vi "Steps Handler.vi"(7 "Operation":enum16{"Setup", "Next State"}(ring), 9 "Zone Setup Array":cluster{"Zone Selector":string, "Timing":dbl}[](array[cluster]), 10 "Run Selector":bool) -> (2 "Next State":cluster{"Value":T1, "Timing":dbl})   [LabVIEW 2025]
uses:
  Controls/States.ctl
panel:
  out "Array 2":cluster{"Value":T1, "Timing":dbl}[](array[cluster])
  out "Array":cluster{"Value":T1, "Timing":dbl}[](array[cluster])
  in  "State":T1
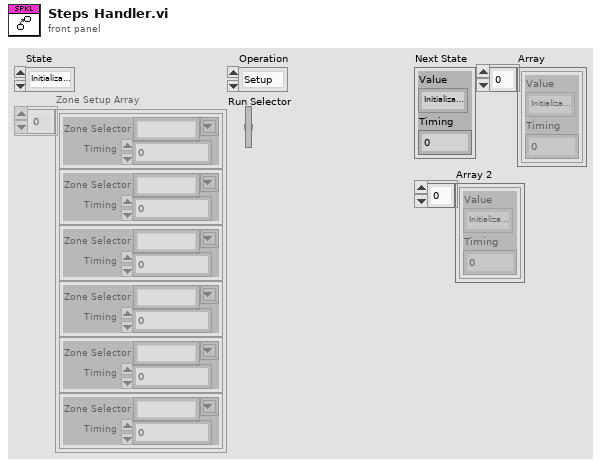
[diagram p1: front panel]
types:
  T1 = typedef "States.ctl" = enum16{"Initialization", "Wait For Start", "Setup", "Sprinkling Program", "North", "East", "South", "West", "Rain", "Low Water"}
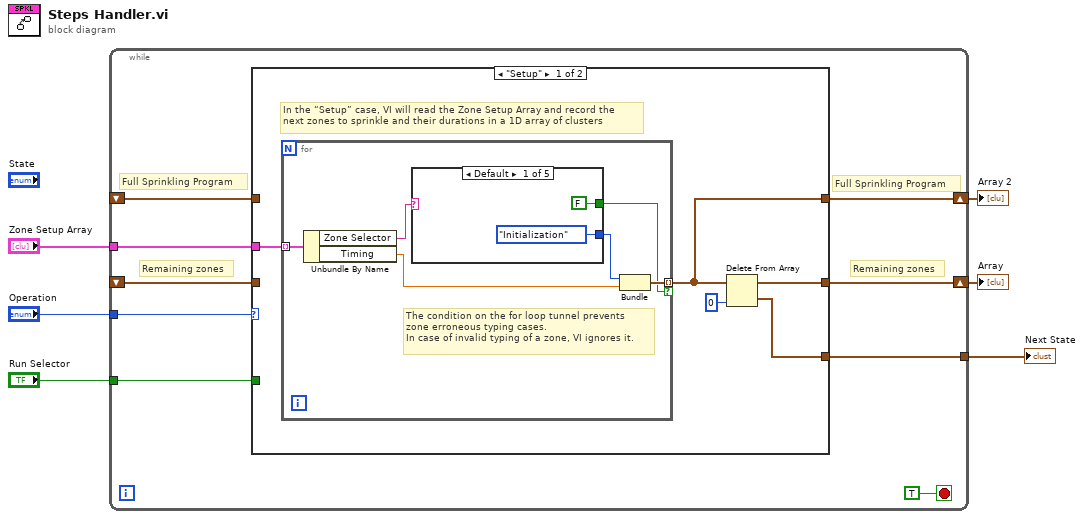
[diagram p0: block diagram]
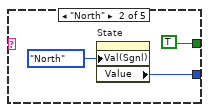
[diagram p2: hidden frame]
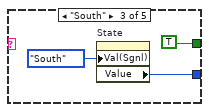
[diagram p3: hidden frame]
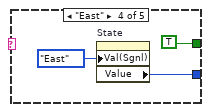
[diagram p4: hidden frame]
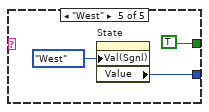
[diagram p5: hidden frame]
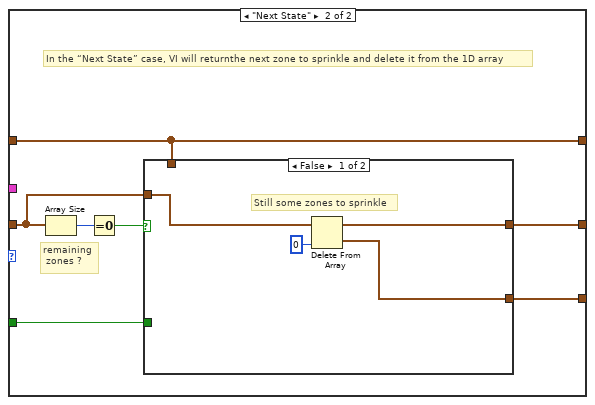
[diagram p6: hidden frame]
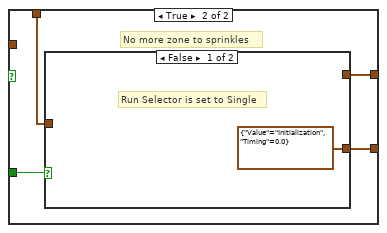
[diagram p7: hidden frame]
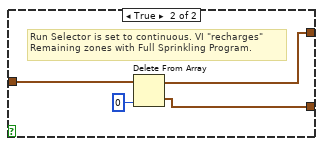
[diagram p8: hidden frame]
diagram:
  n1 = while {
    tunnel: "Operation" -> [w15]
    tunnel: "Zone Setup Array" -> [w13]
    tunnel: [w10] -> w4
    shift-right: [w11] -> w2
    shift-left: _ -> [w8]
    shift-right: [w12] -> w1
    shift-left: _ -> [w9]
    tunnel: "Run Selector" -> [w7]
    stop <- TRUE stop-if-true
    # "Remaining zones"
    # "Full Sprinkling Program"
    # "Remaining zones"
    # "Full Sprinkling Program"
    n2 = case shown="\"Setup\"" w15 {
      tunnel: w13 -> [w20 _]
      tunnel: [w18 w44] -> w12
      tunnel: [w17 w43] -> w11
      tunnel: [w16 w42] -> w10
      tunnel: w9 -> [_ w44]
      tunnel: w8 -> [_ w41]
      tunnel: w7 -> [_ w45]
      frame "Setup" {
        # "In the “Setup” case, VI will read the Zone Setup Array and record the \nnext zones to sprinkle and their durations in a 1D array of clusters"
        n3 = for {
          tunnel: w20 -> [w26] mode=indexing
          tunnel: [w22] -> w18 mode=indexing if=w21
          # "The condition on the for loop tunnel prevents \nzone erroneous typing cases.\nIn case of invalid typing of a zone, VI ignores it."
          n4 = Unbundle By Name(w26) -> ("Zone Selector"=w25:string, "Timing"=w23:dbl)
          n5 = case shown="Default" w25 {
            tunnel: [States."Initialization" ("Value") w30 w33 w36 w39] -> w24
            tunnel: [FALSE TRUE TRUE TRUE TRUE] -> w21
            frame Default {
            }
            frame "North" {
              n6 = property on="State" class="Enum (strict)"("Val(Sgnl)"=States."North" ("Value (Signaling)")) -> ("Value"=w30:T1)  [unwired: 2 in, 2 out]
            }
            frame "South" {
              n7 = property on="State" class="Enum (strict)"("Val(Sgnl)"=States."South" ("Value (Signaling)")) -> ("Value"=w33:T1)  [unwired: 2 in, 2 out]
            }
            frame "East" {
              n8 = property on="State" class="Enum (strict)"("Val(Sgnl)"=States."East" ("Value (Signaling)")) -> ("Value"=w36:T1)  [unwired: 2 in, 2 out]
            }
            frame "West" {
              n9 = property on="State" class="Enum (strict)"("Val(Sgnl)"=States."West" ("Value (Signaling)")) -> ("Value"=w39:T1)  [unwired: 2 in, 2 out]
            }
          }
          n10 = Bundle("Value"=w24, "Timing"=w23) -> (w22:cluster{"Value":T1, "Timing":dbl})  [unwired: 1 in]
        }
        n11 = Delete From Array(array=w18, index=0) -> (deleted portion=w16:cluster{"Value":T1, "Timing":dbl}, array with subset deleted=w17:cluster{"Value":T1, "Timing":dbl}[])  [unwired: 1 in]
      }
      frame "Next State" {
        # "remaining\n zones ?"
        # "In the “Next State” case, VI will returnthe next zone to sprinkle and delete it from the 1D array"
        n12 = Array Size(array=w41) -> (size(s)=w47:i32)
        n13 = Equal To 0?(x=w47) -> (x = 0?=w46:bool)
        n14 = case shown="False" w46 {
          tunnel: w45 -> [_ w55]
          tunnel: w44 -> [_ w54]
          tunnel: [w50 w53] -> w43
          tunnel: [w49 w52] -> w42
          tunnel: w41 -> [w51 _]
          frame False {
            # "Still some zones to sprinkle"
            n15 = Delete From Array(array=w51, index=0) -> (deleted portion=w49:cluster{"Value":T1, "Timing":dbl}, array with subset deleted=w50:cluster{"Value":T1, "Timing":dbl}[])  [unwired: 1 in]
          }
          frame True {
            # "No more zone to sprinkles"
            n16 = case shown="False" w55 {
              tunnel: w54 -> [_ w60]
              tunnel: [_ w58] -> w53
              tunnel: [cluster{"Value":T1, "Timing":dbl} {"Value"=enum."Initialization", "Timing"=0.0} w57] -> w52
              frame False {
                # "Run Selector is set to Single"
              }
              frame True {
                # "Run Selector is set to continuous. VI \"recharges\" \nRemaining zones with Full Sprinkling Program."
                n17 = Delete From Array(array=w60, index=0) -> (deleted portion=w57:cluster{"Value":T1, "Timing":dbl}, array with subset deleted=w58:cluster{"Value":T1, "Timing":dbl}[])  [unwired: 1 in]
              }
            }
          }
        }
      }
    }
  }
  "Next State" <- w4
  "Array" <- w2
  "Array 2" <- w1
